vi "Populate Control.vi"() -> ()   [LabVIEW 2013]
uses:
  lightfield-automation-labview/LightField Automation.lvclass
  C:/Program Files/Princeton Instruments/LightField/PrincetonInstruments.LightFieldAddInSupportServices.dll
  Program Files/Princeton Instruments/LightField/PrincetonInstruments.LightFieldAddInSupportServices.dll
panel:
  in  "Experiment Name":string
  in  "stop":bool
  in  "ADC Quality (Ring Control I32 Representation)":i32(ring)
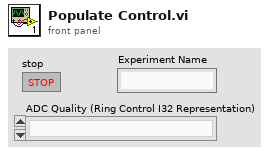
[diagram p1: front panel]
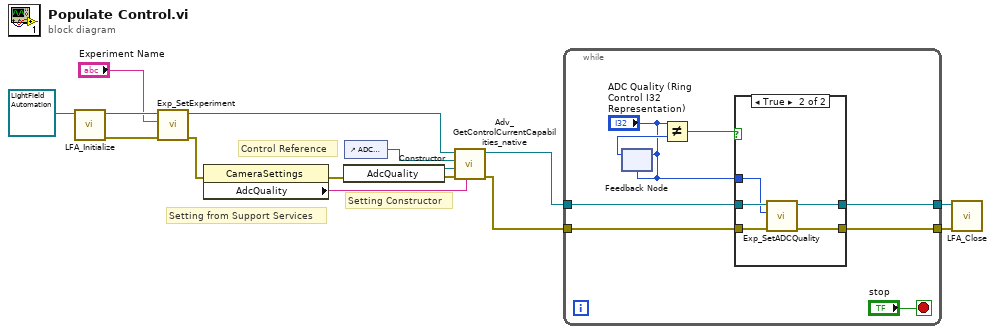
[diagram p0: block diagram]
diagram:
  # "Control Reference"
  # "Setting Constructor"
  # "Setting from Support Services"
  n1 = call "LFA_Initialize.vi"("LightField Automation in"=refnum<class "LightField Automation.lvclass"> refnum ("LightField Automation.lvclass")) -> ("error out"=w6:errorcluster, "LightField Automation out"=w7:refnum<class "LightField Automation.lvclass">)  [unwired: 9 in]
  n2 = call "Exp_SetExperiment.vi"("error in (no error)"=w6, "ExperimentName"="Experiment Name", "LightField Automation in"=w7) -> ("error out"=w3:errorcluster, "LightField Automation out"=w4:refnum<class "LightField Automation.lvclass">)  [unwired: 7 in]
  n3 = property class="CameraSettings"(error in=w3) -> (error out=w11:errorcluster, "AdcQuality"=w13:string)  [unwired: 1 in, 1 out]
  n4 = constructor class="AdcQuality"(error in=w11) -> (reference out=w15:refnum<k24>, error out=w12:errorcluster)  [unwired: 2 in, 1 out]
  n5 = control-ref of="ADC Quality (Ring Control I32 Representation)"() -> (w14:refnum<vi>)
  n6 = call "Adv_GetControlCurrentCapabilities_native.vi"("LightField Setting"=w13, "error in (no error)"=w12, "Enum Class"=w15, "Control"=w14, "LightField Automation in"=w4) -> ("error out"=w9:errorcluster, "LightField Automation out"=w10:refnum<class "LightField Automation.lvclass">)  [unwired: 5 in]
  n7 = while {
    tunnel: w10 -> [w20]
    tunnel: w9 -> [w19]
    tunnel: [w17] -> w1
    tunnel: [w16] -> w2
    stop <- "stop" stop-if-true
    n8 = feedback-in #1("ADC Quality (Ring Control I32 Representation)") -> ()
    n9 = feedback #1("ADC Quality (Ring Control I32 Representation)") -> (w22:i32)
    n10 = Not Equal?(x="ADC Quality (Ring Control I32 Representation)", y=w22) -> (x != y?=w21:bool)
    n11 = case shown="True" w21 {
      tunnel: w20 -> [w25 w30]
      tunnel: w19 -> [w24 w29]
      tunnel: "ADC Quality (Ring Control I32 Representation)" -> [_ w28]
      tunnel: [w25 w27] -> w17
      tunnel: [w24 w26] -> w16
      frame False {
      }
      frame True {
        n12 = call "Exp_SetADCQuality.vi"("error in (no error)"=w29, "ADCQuality"=w28, "LightField Automation in"=w30) -> ("error out"=w26:errorcluster, "LightField Automation out"=w27:refnum<class "LightField Automation.lvclass">)  [unwired: 7 in]
      }
    }
  }
  n13 = call "LFA_Close.vi"("error in (no error)"=w2, "LightField Automation in"=w1) -> ()  [unwired: 8 in, 2 out]
